vi "mes~产品加工参数采集.vi"(8 "error in (no error)":errorcluster caption="错误输入（无错误）", 9 "采集项":string[](array[string]), 11 "测试结果":string caption="测试结果:") -> (0 "error out":errorcluster caption="错误输出", 1 "ErrorMessage":string, 2 "加工参数采集成功":bool)   [LabVIEW 2015]
uses:
  Global.vi
  ctl/SendproductParaColloctUniversal.ctl
  ctl/ReceiveproductParaColloctUniversal.ctl
panel:
  in  "Headers":string[][](array[string])=[["Content-Type", "text/xml;charset=UTF-8"], ["SOAPAction", "\"http://tempuri.org/ICalbProductParaColloctUniversalWcf/productParaColloctUniversal\""], ["Connection", "Keep-Alive"], ["User-Agent", "Apache-HttpClient/4.1.1 (java 1.5)"]]
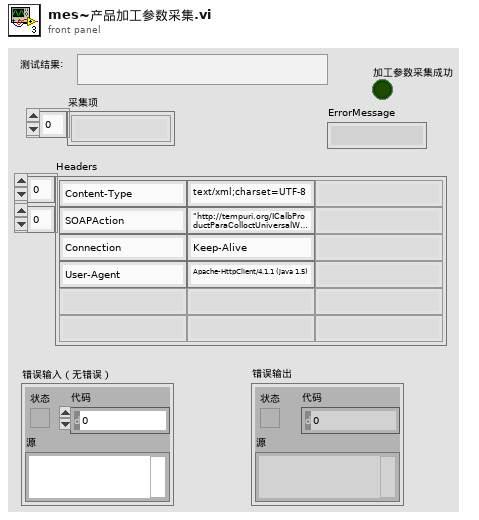
[diagram p1: front panel]
types:
  T1 = typedef "SendproductParaColloctUniversal.ctl" = cluster{"#attributes":cluster{"xmlns:soapenv":string, "xmlns:tem":string, "xmlns:cal":string}, "soapenv:Header":string, "soapenv:Body":cluster{"tem:productParaColloctUniversal":cluster{"tem:vo":cluster{"cal:completeQty":string, "cal:equipNum":string, "cal:identification":string, "cal:productType":string, "cal:qualityStatus":string, "cal:recordDate":string, "cal:siteCode":string, "cal:tagData":cluster{"cal:TagDataVO":cluster{"cal:tagCode":string, "cal:tagValue":string}[]}, "cal:testOrderNum":string, "cal:userName":string}}}}
  T2 = cluster{"接口地址(URL)":string, "权限校验":string, "产品进站":string, "参数采集":string, "产品出站":string, "设备状态":string, "设备编号(equipNum)":string, "站点名称(siteCode)":string, "生产类型(productType)":string, "试验单号(testOrderNum)":string}
  T3 = typedef "ReceiveproductParaColloctUniversal.ctl" = cluster{"#attributes":cluster{"xmlns:s":string}, "s:Body":cluster{"productParaColloctUniversalResponse":cluster{"#attributes":cluster{"xmlns":string}, "productParaColloctUniversalResult":cluster{"#attributes":cluster{"xmlns:a":string, "xmlns:i":string}, "a:ErrorCode":string, "a:ErrorMessage":string, "a:Success":string}}}}
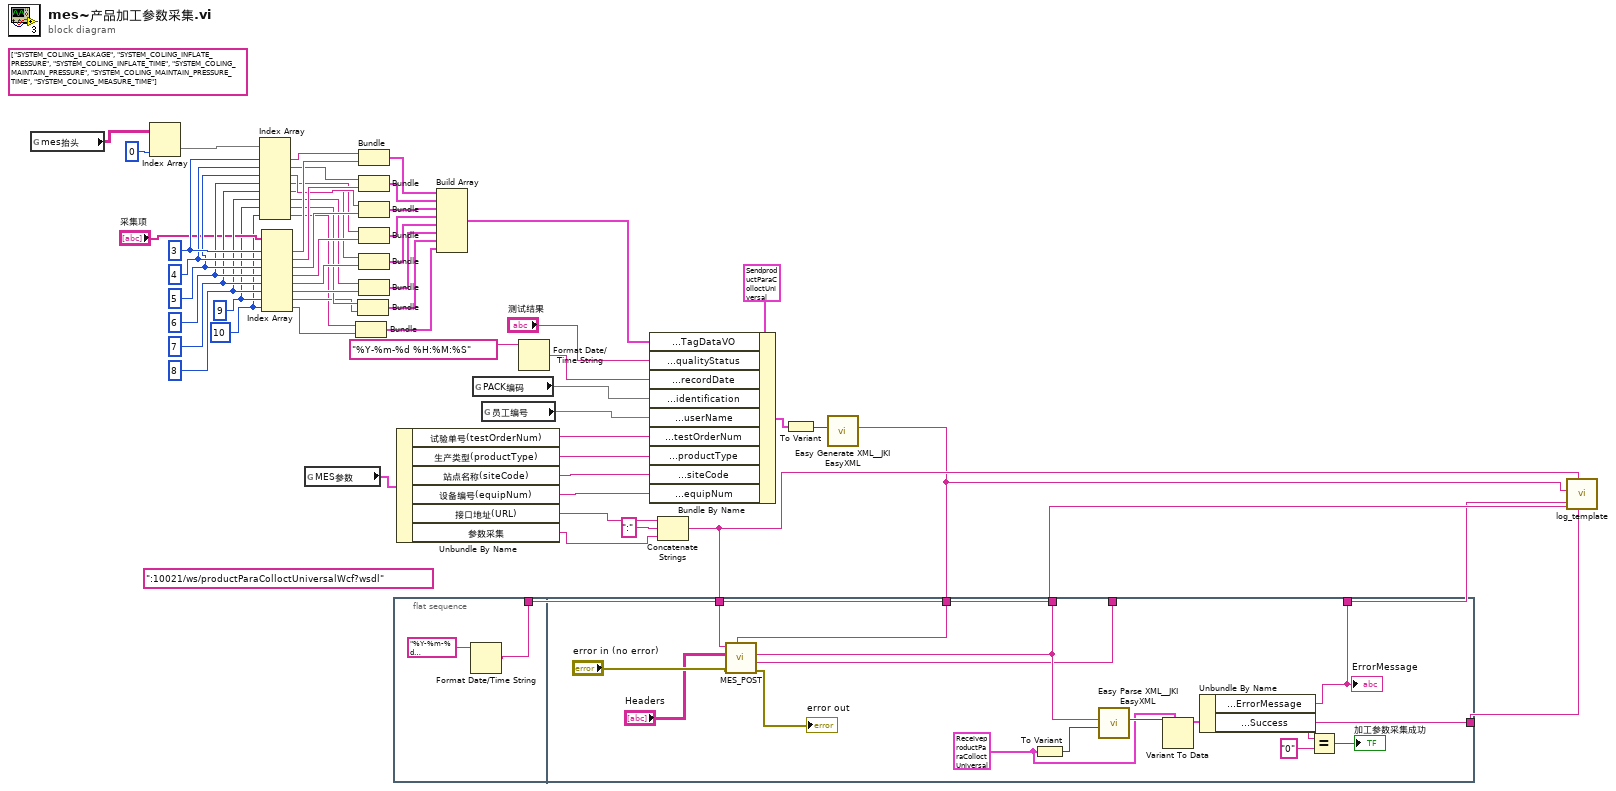
[diagram p0: block diagram]
diagram:
  w12 = 10 ("索引")
  w13 = 9 ("索引")
  (unwired) string[] ["SYSTEM_COLING_LEAKAGE", "SYSTEM_COLING_INFLATE_PRESSURE", "SYSTEM_COLING_INFLATE_TIME", "SYSTEM_COLING_MAINTAIN_PRESSURE", "SYSTEM_COLING_MAINTAIN_PRESSURE_TIME", "SYSTEM_COLING_MEASURE_TIME"]
  w18 = 8 ("索引")
  w20 = 7 ("索引")
  w21 = 6 ("索引")
  w22 = 5 ("索引")
  w23 = 4 ("索引")
  w24 = 3 ("索引")
  (unwired) ":10021/ws/productParaColloctUniversalWcf?wsdl"
  n1 = global read "Global.vi" "mes抬头"() -> (w26:string[][])
  n2 = Index Array(array=w26, index (col)=0 ("禁用的索引 (列)")) -> (element=w25:string[])  [unwired: 1 in]
  n3 = Index Array(array=w25, index #1=w24, index #2=w23, index #3=w22, index #4=w21, index #5=w20, index #6=w18, index #7=w13, index #8=w12) -> (element #1=w42:string, element #2=w41:string, element #3=w40:string, element #4=w38:string, element #5=w36:string, element #6=w34:string, element #7=w11:string, element #8=w9:string)
  n4 = Index Array(array="采集项", index #1=w24, index #2=w23, index #3=w22, index #4=w21, index #5=w20, index #6=w18, index #7=w13, index #8=w12) -> (element #1=w44:string, element #2=w43:string, element #3=w39:string, element #4=w37:string, element #5=w35:string, element #6=w33:string, element #7=w10:string, element #8=w8:string)
  n5 = global read "Global.vi" "MES参数"() -> (w54:T2)
  n6 = Bundle("String"=w9, "值解析"=w8) -> (w6:cluster{"String":string, "值解析":string})  [unwired: 1 in]
  n7 = Bundle("String"=w11, "值解析"=w10) -> (w7:cluster{"String":string, "值解析":string})  [unwired: 1 in]
  n8 = Bundle("String"=w42, "值解析"=w44) -> (w51:cluster{"String":string, "值解析":string})  [unwired: 1 in]
  n9 = Bundle("String"=w41, "值解析"=w43) -> (w32:cluster{"String":string, "值解析":string})  [unwired: 1 in]
  n10 = Bundle("String"=w40, "值解析"=w39) -> (w31:cluster{"String":string, "值解析":string})  [unwired: 1 in]
  n11 = Bundle("String"=w38, "值解析"=w37) -> (w30:cluster{"String":string, "值解析":string})  [unwired: 1 in]
  n12 = Bundle("String"=w36, "值解析"=w35) -> (w29:cluster{"String":string, "值解析":string})  [unwired: 1 in]
  n13 = Bundle("String"=w34, "值解析"=w33) -> (w19:cluster{"String":string, "值解析":string})  [unwired: 1 in]
  n14 = flat-sequence {
    tunnel: [w59] -> w3
    tunnel: w4 -> [w66]
    tunnel: [w65] -> _
    tunnel: w5 -> [w67]
    tunnel: [w64] -> _
    tunnel: [w62] -> w1
    tunnel: [w61] -> w2
    frame #0 {
      n15 = Format Date/Time String(time format string (%c)="%Y-%m-%d %H:%M:%S%3u-->" ("EndTime")) -> (date/time string=w59:string)  [unwired: 2 in]
    }
    frame #1 {
      w70 = T3 {"#attributes"={"xmlns:s"="http://schemas.xmlsoap.org/soap/envelope/"}, "s:Body"={"productParaColloctUniversalResponse"={"#attributes"={"xmlns"="http://tempuri.org/"}, "productParaColloctUniversalResult"={"#attributes"={"xmlns:a"="http://schemas.datacontract.org/2004/07/EdgeUtility", "xmlns:i"="http://www.w3.org/2001/XMLSchema-instance"}, "a:ErrorCode"="", "a:ErrorMessage"="", "a:Success"=""}}}} ("s:Envelope")
      n16 = call "MES_POST.vi"("DATA"=w66, "错误输入（无错误）"="error in (no error)", 10:"Headers", "URL"=w67) -> ("错误输出"=→"error out":errorcluster, "headers"=w64:string, "body"=w65:string)  [unwired: 5 in]
      n17 = To Variant(anything=w70) -> (Variant=w75:variant)
      n18 = call <vilib>:"Easy Parse XML__JKI EasyXML.vi"("LabVIEW Data (Type)"=w75, "XML String"=w65) -> ("LabVIEW Data"=w74:variant)  [unwired: 8 in, 1 out]
      n19 = Variant To Data(type=w70, Variant=w74) -> (data=w73:T3)  [unwired: 1 in, 1 out]
      n20 = Unbundle By Name(w73) -> ("s:Body.productParaColloctUniversalResponse.productParaColloctUniversalResult.a:ErrorMessage"=w62:string, "s:Body.productParaColloctUniversalResponse.productParaColloctUniversalResult.a:Success"=w61:string)
      "ErrorMessage" <- w62
      n21 = Equal?(x=w61, y="0") -> (x = y?=→"加工参数采集成功":bool)
    }
  }
  n22 = Unbundle By Name(w54) -> ("试验单号(testOrderNum)"=w50:string, "生产类型(productType)"=w52:string, "站点名称(siteCode)"=w55:string, "设备编号(equipNum)"=w56:string, "接口地址(URL)"=w53:string, "参数采集"=w15:string)
  n23 = Build Array(w51, w32, w31, w30, w29, w19, w7, w6) -> (w28:cluster{"String":string, "值解析":string}[])
  n24 = global read "Global.vi" "PACK编码"() -> (w48)
  n25 = global read "Global.vi" "员工编号"() -> (w49)
  n26 = Format Date/Time String(time format string (%c)="%Y-%m-%d %H:%M:%S" ("时间格式字符串(%c)")) -> (date/time string=w46:string)  [unwired: 2 in]
  n27 = Bundle By Name(cluster=T1 {"#attributes"={"xmlns:soapenv"="http://schemas.xmlsoap.org/soap/envelope/", "xmlns:tem"="http://tempuri.org/", "xmlns:cal"="http://schemas.datacontract.org/2004/07/CalbProductParaColloctUniversalService"}, "soapenv:Header"="", "soapenv:Body"={"tem:productParaColloctUniversal"={"tem:vo"={"cal:completeQty"="", "cal:equipNum"="", "cal:identification"="", "cal:productType"="", "cal:qualityStatus"="", "cal:recordDate"="", "cal:siteCode"="", "cal:tagData"={"cal:TagDataVO"=[]}, "cal:testOrderNum"="", "cal:userName"=""}}}} ("soapenv:Envelope"), "soapenv:Body.tem:productParaColloctUniversal.tem:vo.cal:tagData.cal:TagDataVO"=w28, "soapenv:Body.tem:productParaColloctUniversal.tem:vo.cal:qualityStatus"="测试结果", "soapenv:Body.tem:productParaColloctUniversal.tem:vo.cal:recordDate"=w46, "soapenv:Body.tem:productParaColloctUniversal.tem:vo.cal:identification"=w48, "soapenv:Body.tem:productParaColloctUniversal.tem:vo.cal:userName"=w49, "soapenv:Body.tem:productParaColloctUniversal.tem:vo.cal:testOrderNum"=w50, "soapenv:Body.tem:productParaColloctUniversal.tem:vo.cal:productType"=w52, "soapenv:Body.tem:productParaColloctUniversal.tem:vo.cal:siteCode"=w55, "soapenv:Body.tem:productParaColloctUniversal.tem:vo.cal:equipNum"=w56) -> (w58:T1)
  n28 = Concatenate Strings(w53, ":" ("字符串"), w15) -> (w5:string)
  n29 = To Variant(anything=w58) -> (Variant=w57:variant)
  n30 = call <vilib>:"Easy Generate XML__JKI EasyXML.vi"("LabVIEW Data"=w57) -> ("XML String"=w4:string)  [unwired: 9 in, 1 out]
  n31 = call "log_template.vi"(4:w1, 6:w2, 7:w5, 8:w3, 10:w4) -> ()  [unwired: 7 in]
